vi "Soft Panel.vi"(8 "error in (no error)":errorcluster, 11 "JMETestSolutions.Instrument in":refnum<class "JMETestSolutions.Instrument.lvclass">) -> (0 "error out":errorcluster, 3 "JMETestSolutions.Instrument out":refnum<class "JMETestSolutions.Instrument.lvclass">)   [LabVIEW 2020, in "JMETestSolutions.Instrument.lvlib" / "JMETestSolutions.Instrument.lvclass"]
doc: "Soft Panels are used to control and test the Instrument"
uses:
  JMETestSolutions.Instrument.lvclass
panel:
  in  "stop":bool
  # "Base Insturment Class Soft Panel"
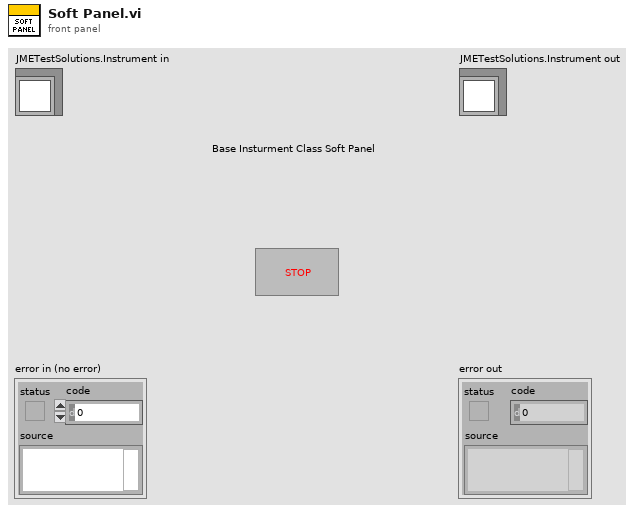
[diagram p1: front panel]
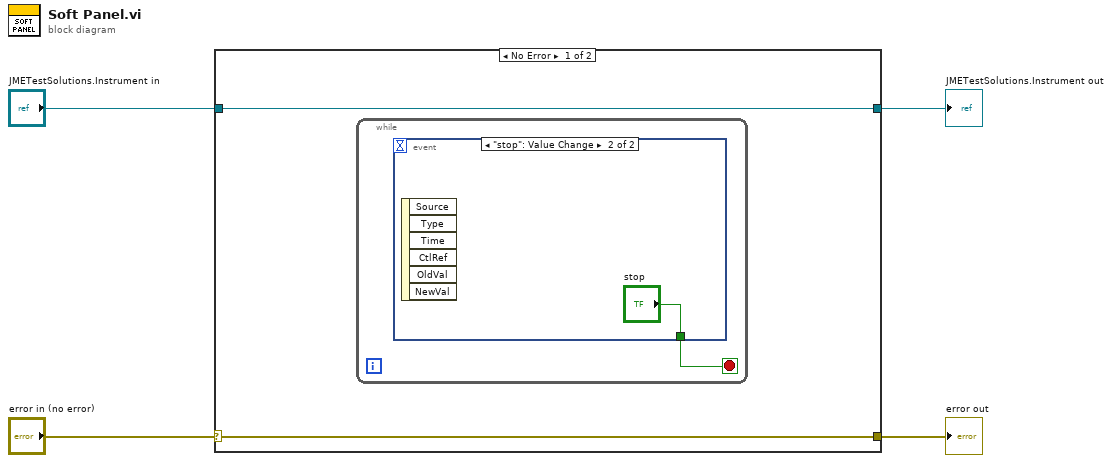
[diagram p0: block diagram]
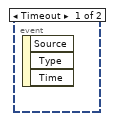
[diagram p2: hidden frame]
diagram:
  n1 = case shown="No Error" "error in (no error)" {
    selector: "error in (no error)" -> [w5 w10]
    tunnel: [w5 w10] -> w3
    tunnel: [w6 w9] -> w1
    tunnel: "JMETestSolutions.Instrument in" -> [w6 w9]
    frame No Error {
      n2 = while {
        stop <- w7 stop-if-true
        n3 = event shown="[1] \"stop\": Value Change" {
          selector: _ -> [_ _]
          dyn-events: _ -> [_ _]
          timeout: _ -> [_ _]
          tunnel: [_ "stop"] -> w7
          event Timeout {
            n4 = event-data() -> ()  [unwired: 1 in, 3 out]
          }
          event "stop": Value Change {
            n5 = event-data() -> ()  [unwired: 1 in, 6 out]
          }
        }
      }
    }
    frame Error {
    }
  }
  "error out" <- w3
  "JMETestSolutions.Instrument out" <- w1
